vi "Edit Data.vi"(2 "error in (no error)":errorcluster, 3 "History Data input":T2) -> (0 "error out":errorcluster, 1 "History Data output":T2)   [LabVIEW 2021]
doc: "Este VI se encarga de editar/recortar los datos de temperatura"
panel:
  in  "Edit button":bool
  in  "Posicion final":dbl min=0.0 step=0.5
  in  "Posicion inicial":dbl min=0.0 step=0.5
  out "Temperature Data":T1(graph)=[{"Temp.Max"=27.3, "Temp.Actual"=25.6276741088368, "Temp.Min"=27.1}, {"Temp.Max"=27.3, "Temp.Actual"=25.73080566013232, "Temp.Min"=27.1}, {"Temp.Max"=27.3, "Temp.Actual"=25.74369710404426, "Temp.Min"=27.1}, {"Temp.Max"=27.3, "Temp.Actual"=25.74369710404426, "Temp.Min"=27.1}, {"Temp.Max"=27.3, "Temp.Actual"=25.74369710404426, "Temp.Min"=27.1}, {"Temp.Max"=27.3, "Temp.Actual"=25.74369710404426, "Temp.Min"=27.1}, {"Temp.Max"=27.3, "Temp.Actual"=25.846828655339777, "Temp.Min"=27.3}, {"Temp.Max"=27.3, "Temp.Actual"=25.885502987075597, "Temp.Min"=27.3}, {"Temp.Max"=27.3, "Temp.Actual"=25.898394430987537, "Temp.Min"=27.3}, {"Temp.Max"=27.3, "Temp.Actual"=25.898394430987537, "Temp.Min"=27.3}, {"Temp.Max"=30.3, "Temp.Actual"=25.937068762723356, "Temp.Min"=27.3}, {"Temp.Max"=30.3, "Temp.Actual"=26.001525982283056, "Temp.Min"=27.3}, {"Temp.Max"=30.3, "Temp.Actual"=26.014417426194996, "Temp.Min"=27.3}, {"Temp.Max"=30.3, "Temp.Actual"=26.040200314018875, "Temp.Min"=27.3}, {"Temp.Max"=27.3, "Temp.Actual"=26.065983201842755, "Temp.Min"=27.3}, {"Temp.Max"=27.3, "Temp.Actual"=26.130440421402454, "Temp.Min"=27.3}, {"Temp.Max"=27.3, "Temp.Actual"=26.156223309226334, "Temp.Min"=27.3}, {"Temp.Max"=27.3, "Temp.Actual"=26.182006197050214, "Temp.Min"=27.3}, {"Temp.Max"=27.3, "Temp.Actual"=26.233571972697973, "Temp.Min"=26.3}, {"Temp.Max"=27.3, "Temp.Actual"=26.285137748345733, "Temp.Min"=25.3}, {"Temp.Max"=27.3, "Temp.Actual"=26.272246304433793, "Temp.Min"=25.3}, {"Temp.Max"=27.3, "Temp.Actual"=26.272246304433793, "Temp.Min"=25.3}, {"Temp.Max"=27.3, "Temp.Actual"=26.336703523993492, "Temp.Min"=25.3}, {"Temp.Max"=30.3, "Temp.Actual"=26.362486411817372, "Temp.Min"=25.3}, {"Temp.Max"=30.3, "Temp.Actual"=26.41405218746513, "Temp.Min"=25.3}, {"Temp.Max"=30.3, "Temp.Actual"=26.43983507528901, "Temp.Min"=25.3}, {"Temp.Max"=30.3, "Temp.Actual"=26.46561796311289, "Temp.Min"=25.3}]
  # "Elige con que tramo quedarte y toma pasos múltiplos de 0,5"
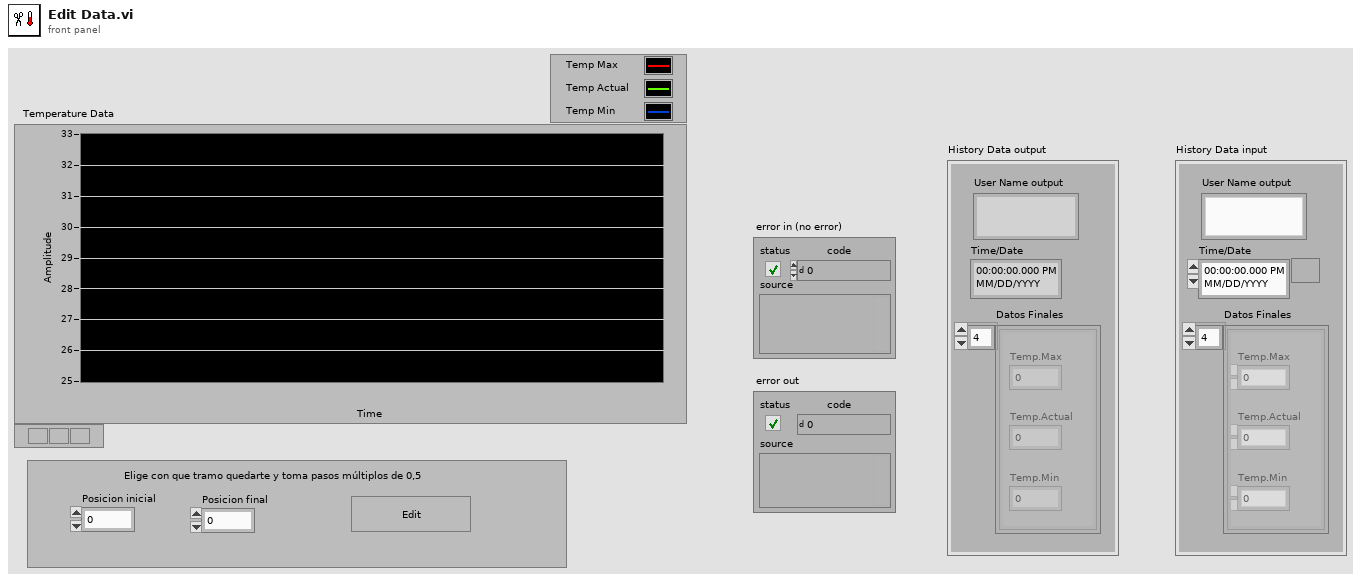
[diagram p1: front panel]
types:
  T1 = cluster{"Temp.Max":dbl, "Temp.Actual":dbl, "Temp.Min":dbl}[]
  T2 = cluster{"User Name output":string, "Time/Date":timestamp, "Datos Finales":cluster{"Temp.Max":dbl, "Temp.Actual":dbl, "Temp.Min":dbl}[]}
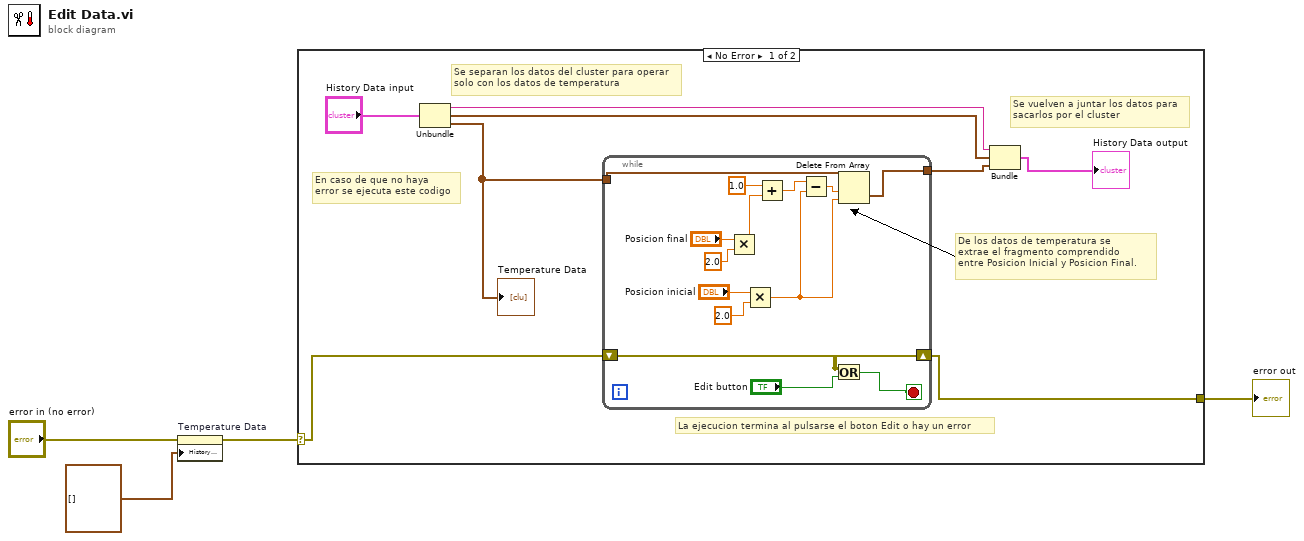
[diagram p0: block diagram]
diagram:
  n1 = property on="Temperature Data" class="WFChart (strict)"(error in="error in (no error)", "History Data"=T1 []) -> (error out=w1:errorcluster)  [unwired: 1 in, 1 out]
  n2 = case shown="No Error" w1 {
    selector: w1 -> [w6 w27]
    tunnel: [w5 w27] -> w4
    frame No Error {
      # "La ejecucion termina al pulsarse el boton Edit o hay un error"
      # "Se vuelven a juntar los datos para\nsacarlos por el cluster"
      # "De los datos de temperatura se \nextrae el fragmento comprendido\nentre Posicion Inicial y Posicion Final."
      # "Se separan los datos del cluster para operar\nsolo con los datos de temperatura"
      # "En caso de que no haya\nerror se ejecuta este codigo"
      n3 = Unbundle("History Data input") -> ("User Name output"=w8:string, "Time/Date"=w9:timestamp, "Datos Finales"=w10:T1)
      "Temperature Data" <- w10
      n4 = while {
        tunnel: w10 -> [w20]
        tunnel: [w16] -> w11
        shift-right: [w19] -> w5
        shift-left: w6 -> [w19]
        stop <- w21 stop-if-true
        n5 = Multiply(x="Posicion final", y=2.0) -> (x*y=w14:dbl)
        n6 = Multiply(x="Posicion inicial", y=2.0) -> (x*y=w18:dbl)
        n7 = Add(x=1.0, y=w14) -> (x+y=w15:dbl)
        n8 = Subtract(x=w15, y=w18) -> (x-y=w17:dbl)
        n9 = Or(x=w19, y="Edit button") -> (x .or. y?=w21:bool)
        n10 = Delete From Array(array=w20, length=w17, index=w18) -> (deleted portion=w16:T1)  [unwired: 1 out]
      }
      n11 = Bundle("User Name output"=w8, "Time/Date"=w9, "Datos Finales"=w11) -> (→"History Data output":T2)  [unwired: 1 in]
    }
    frame Error {
      # "Si llega un error desde fuera de este VI se\npasa directamente"
    }
  }
  "error out" <- w4
